vi "Read dev in px.vi"(8 "error in (no error)":errorcluster, 11 "Analyze BeamDeviation in":refnum<class "Analyze BeamDeviation.lvclass">) -> (0 "error out":errorcluster, 2 "dev in px":bool, 3 "Analyze BeamDeviation out":refnum<class "Analyze BeamDeviation.lvclass">)   [LabVIEW 2020, in "Analyze.lvlib" / "Analyze BeamDeviation.lvclass"]
uses:
  Analyze BeamDeviation.lvclass
  Analyze BeamDeviation.lvclass/Analyze BeamDeviation.ctl
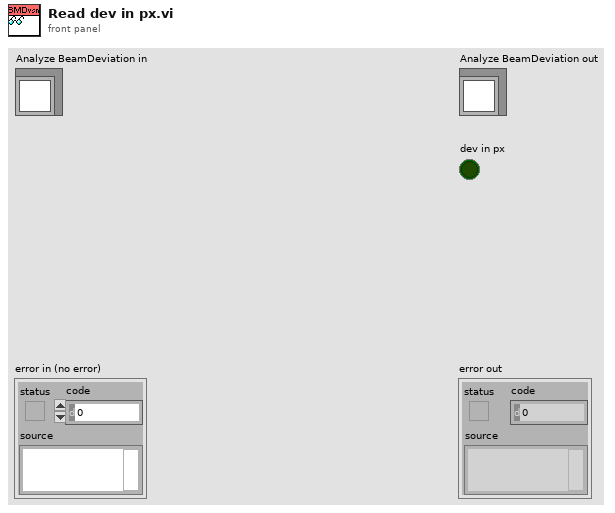
[diagram p1: front panel]
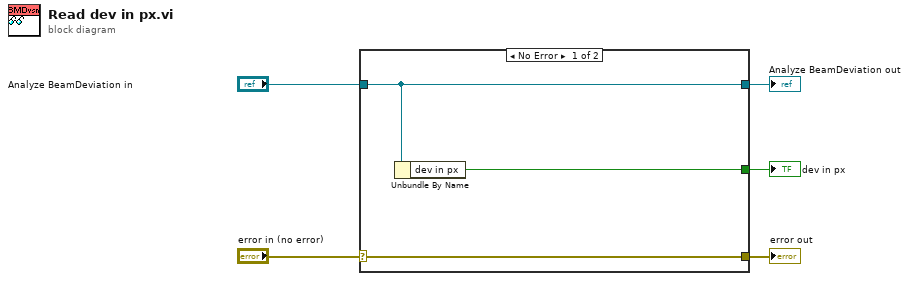
[diagram p0: block diagram]
diagram:
  n1 = case shown="No Error" "error in (no error)" {
    selector: "error in (no error)" -> [w8 w9]
    tunnel: [w8 w9] -> w4
    tunnel: [w7 w10] -> w2
    tunnel: "Analyze BeamDeviation in" -> [w7 w10]
    tunnel: [w6 _] -> w1
    frame No Error {
      n2 = Unbundle By Name(w7) -> ("dev in px"=w6:bool)
    }
    frame Error {
    }
  }
  "error out" <- w4
  "Analyze BeamDeviation out" <- w2
  "dev in px" <- w1
